vi "JSON to LVObject - No Data Member - Returns Matching Type.vi"() -> ()   [LabVIEW 2017, in "Generic Object Serializer Tests.lvlib" / "Type Name Handling.lvlib"]
uses:
  Type Name Handling.lvlib
  No Data Member Subclass/No Data Member Subclass.lvclass
  Generic Object Serializer/Generic Object Serializer.lvclass
  Generic Object Serializer/Type Name Handling.ctl
  Generic Object Serializer/Generic Object Serializer.lvclass/Generic Object Serializer.ctl
  Generic Object Serializer/Write Type Name Handling.vi
  <vilib>/addons/_JKI Toolkits/Caraya/classes/Assert/Assert Equal Value_Variant.vi
  <vilib>/addons/_JKI Toolkits/Caraya/classes/Test/Test.lvclass
  <vilib>/addons/_JKI Toolkits/Caraya/classes/Assert/Assert.lvclass
panel:
  out "error out":errorcluster
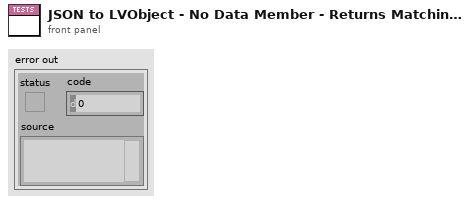
[diagram p1: front panel]
types:
  T1 = typedef "Generic Object Serializer.lvclass/Type Name Handling.ctl" = enum16{"None", "Inline"}
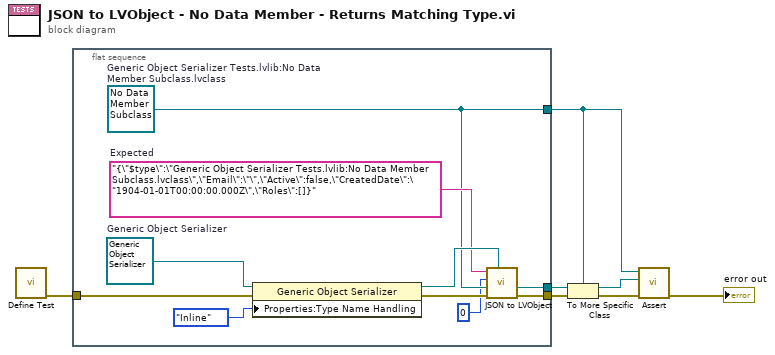
[diagram p0: block diagram]
diagram:
  n1 = call <vilib>:"Define Test.vi"() -> ("error out"=w7:errorcluster)  [unwired: 11 in]
  n2 = flat-sequence {
    tunnel: w7 -> [w13]
    tunnel: [w17] -> w5
    tunnel: [w10] -> w3
    tunnel: [w9] -> w2
    frame #0 {
      w11 = "{\"$type\":\"Generic Object Serializer Tests.lvlib:No Data Member Subclass.lvclass\",\"Email\":\"\",\"Active\":false,\"CreatedDate\":\"1904-01-01T00:00:00.000Z\",\"Roles\":[]}"  # Expected
      w16 = refnum<class "Generic Object Serializer.lvclass"> refnum  # Generic Object Serializer
      w9 = refnum<class "No Data Member Subclass.lvclass"> refnum  # Generic Object Serializer Tests.lvlib:No Data Member Subclass.lvclass
      n3 = property class="Generic Object Serializer"(reference=w16, error in=w13, "Properties:Type Name Handling"=Type_Name_Handling."Inline" ("Type Name Handling")) -> (reference out=w15:refnum<class "Generic Object Serializer.lvclass">, error out=w12:errorcluster)
      n4 = call-dynamic "JSON to LVObject.vi"("LVClass Serializer"=w15, "error in (no error)"=w12, "Object Type"=w9, "Offset"=0, "JSON"=w11) -> ("error out"=w17:errorcluster, "Object"=w10:refnum<class>)  [unwired: 5 in]
    }
  }
  n5 = To More Specific Class(target class=w2, reference=w3, error in=w5) -> (specific class reference=w1:refnum<class "No Data Member Subclass.lvclass">, error out=w4:errorcluster)
  n6 = call-poly <vilib>:"Assert.vi"("error in (no error)"=w4, "Y"=w1, "X"=w2) -> ("error out"=→"error out":errorcluster)  [unwired: 8 in]
